vi "MIMIC_Test.vi"() -> ()   [LabVIEW 2014]
uses:
  Responses/MIMIC_ResponseCluster.ctl
panel:
  in  "Image":bool
  in  "Input_Data":string[](array[string])
  out "Generic_Mimic_Data":T1
  in  "Send":bool
  in  "Command":string
  in  "QUIT":bool
  in  "VISA_IN":refnum<visa-resource-name>="COM4"
  in  "Port Setting":T2={"baud rate"=9600, "data bits"=8, "parity (0:none)"=enum."None", "stop bits (10: 1 bit)"=10} {"stop bits (10: 1 bit)" items=["1.0"=10, "1.5"=15, "2.0"=20]; "data bits" min=5 max=8 step=1}
  out "Error_Out":errorcluster
  in  "Error_In":errorcluster
  # "LIST of Commands:\n1.- EnterFATMode\n2.- ExitFATMode\n3.- SendAck\n4.- StartSession\n5.- ImagerMode"
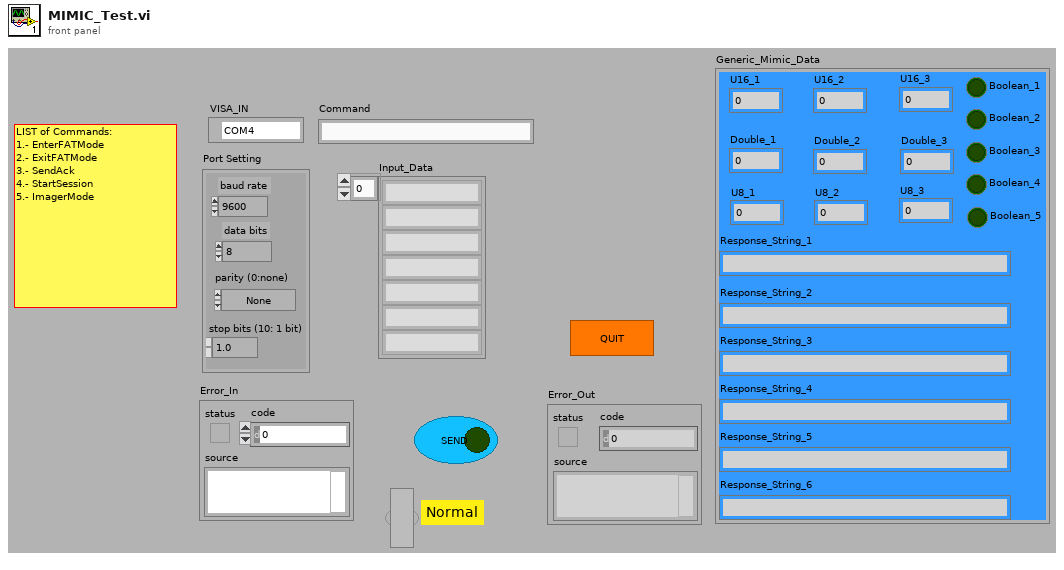
[diagram p1: front panel]
types:
  T1 = typedef "MIMIC_ResponseCluster.ctl" = cluster{"Response_String_1":string, "Response_String_2":string, "Response_String_3":string, "Response_String_4":string, "Response_String_5":string, "Response_String_6":string, "U16_1":u16, "Boolean_1":bool, "Boolean_2":bool, "Boolean_3":bool, "Boolean_4":bool, "Boolean_5":bool, "U16_2":u16, "U16_3":u16, "Double_1":dbl, "Double_2":dbl, "Double_3":dbl, "U8_1":dbl, "U8_2":dbl, "U8_3":dbl}
  T2 = cluster{"baud rate":u32, "data bits":u16, "parity (0:none)":enum16{"None", "Odd", "Even", "Mark", "Space"}, "stop bits (10: 1 bit)":u16}
  T3 = enum16{"OpenPort", "Initial Serial Port", "Write", "ByteRead", "Read", "ClearBuff", "Close"}
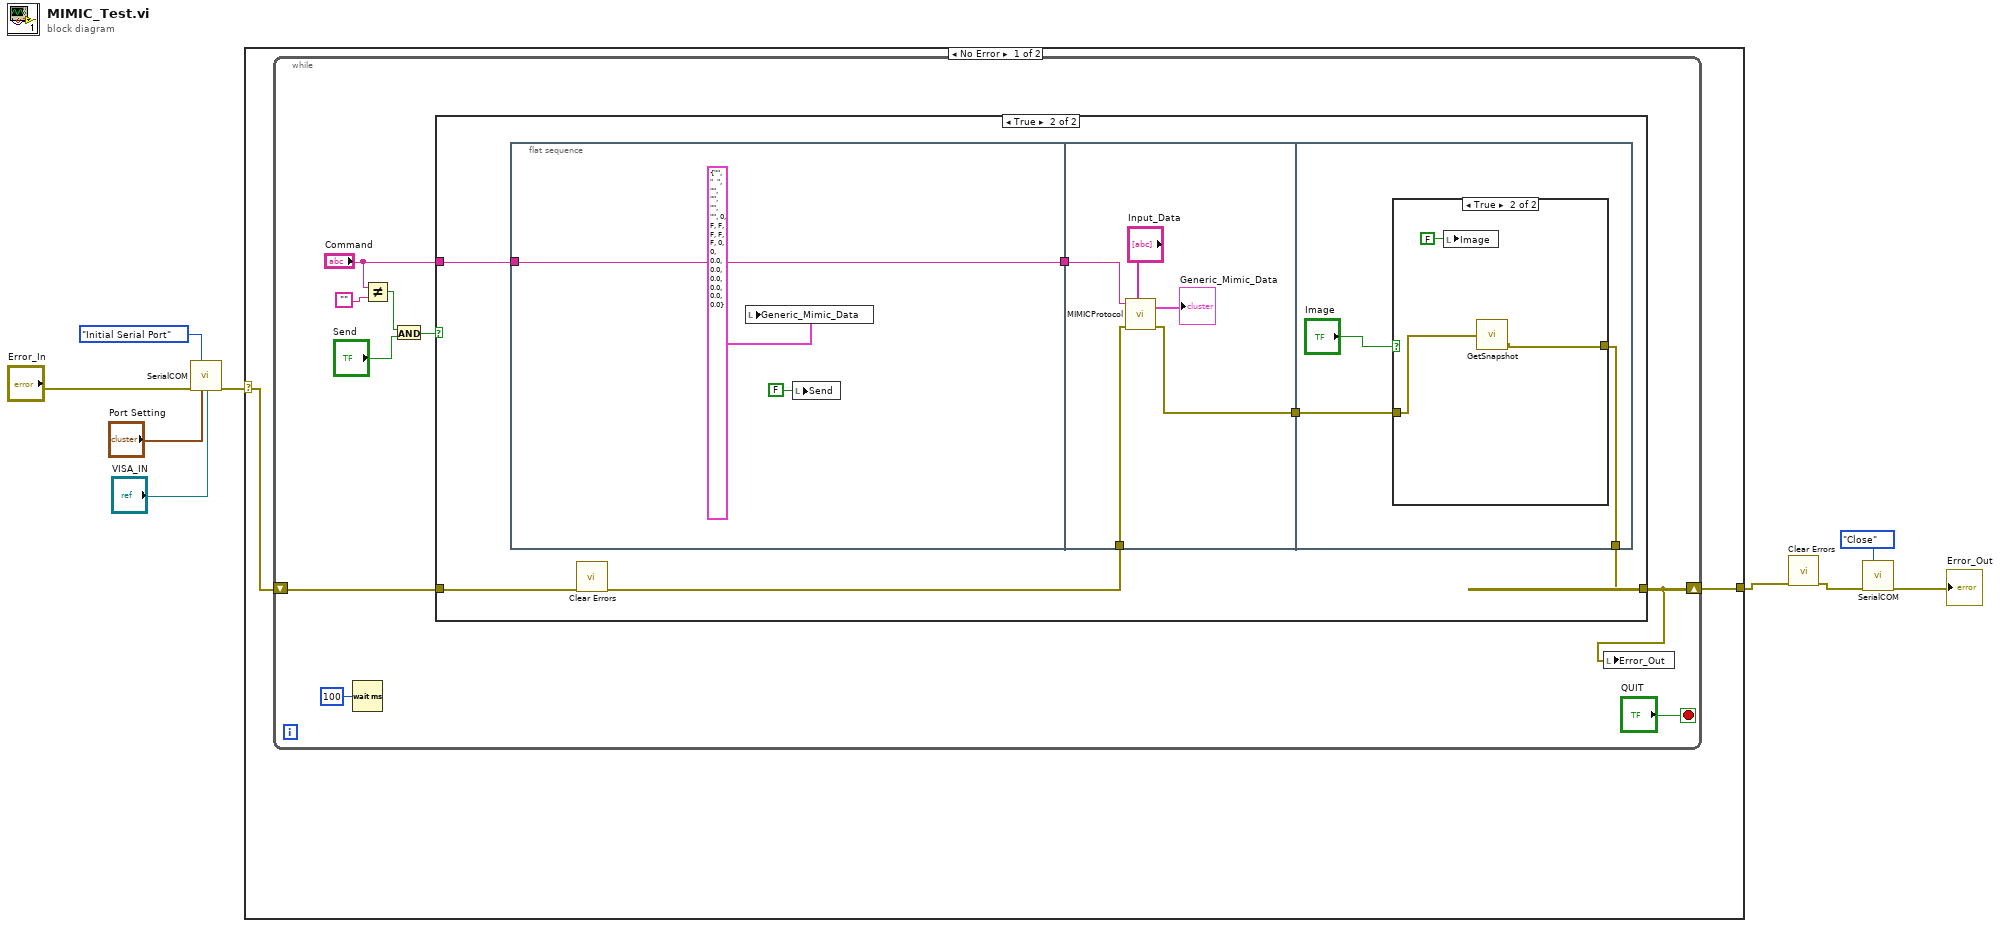
[diagram p0: block diagram]
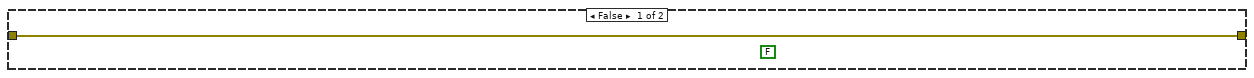
[diagram p2: hidden frame]
diagram:
  n1 = call "SerialCOM.vi"("Function"=T3."Initial Serial Port", "error in (no error)"="Error_In", "Port Setting"="Port Setting", "VISA_IN"="VISA_IN") -> ("error out"=w5:errorcluster)  [unwired: 6 in, 5 out]
  n2 = case shown="No Error" w5 {
    selector: w5 -> [w11 w43]
    tunnel: [w10 w43] -> w2
    frame No Error {
      n3 = while {
        shift-right: [w17] -> w10
        shift-left: w11 -> [w20]
        stop <- "QUIT" stop-if-true
        n4 = Wait (ms)(milliseconds to wait=u32 100) -> ()  [unwired: 1 out]
        n5 = Not Equal?(x="Command", y="") -> (x != y?=w14:bool)
        n6 = And(x=w14, y="Send") -> (x .and. y?=w12:bool)
        n7 = case shown="True" w12 {
          tunnel: w20 -> [w21 w25]
          tunnel: [w21 w22] -> w17
          tunnel: "Command" -> [_ w27]
          frame False {
            (unwired) FALSE
          }
          frame True {
            n8 = flat-sequence {
              tunnel: w27 -> [w30]
              tunnel: [w30] -> w26
              tunnel: w24 -> [w34]
              tunnel: w26 -> [w33]
              tunnel: [w31] -> w23
              tunnel: w23 -> [w37]
              tunnel: [w36] -> w22
              frame #0 {
                n9 = local write "Generic_Mimic_Data"(T1 {"Response_String_1"="", "Response_String_2"="  ", "Response_String_3"="", "Response_String_4"="", "Response_String_5"="", "Response_String_6"="", "U16_1"=0, "Boolean_1"=FALSE, "Boolean_2"=FALSE, "Boolean_3"=FALSE, "Boolean_4"=FALSE, "Boolean_5"=FALSE, "U16_2"=0, "U16_3"=0, "Double_1"=0.0, "Double_2"=0.0, "Double_3"=0.0, "U8_1"=0.0, "U8_2"=0.0, "U8_3"=0.0} ("Generic_Mimic_Data")) -> ()
                n10 = local write "Send"(FALSE ("Send")) -> ()
              }
              frame #1 {
                n11 = call "MIMICProtocol.vi"("Input_Data"="Input_Data", "Error In"=w34, "MIMIC_Command"=w33) -> ("Error Out"=w31:errorcluster, "Generic_Mimic_Data 2"=→"Generic_Mimic_Data":T1)  [unwired: 2 in, 2 out]
              }
              frame #2 {
                n12 = case shown="True" "Image" {
                  tunnel: w37 -> [w39 w41]
                  tunnel: [w39 w40] -> w36
                  frame False {
                  }
                  frame True {
                    n13 = local write "Image"(FALSE ("Image")) -> ()
                    n14 = call "GetSnapshot.vi"("error in"=w41) -> ("error out"=w40:errorcluster)  [unwired: 1 out]
                  }
                }
              }
            }
            n15 = call <vilib>:"Clear Errors.vi"("error in (no error)"=w25) -> ("error out"=w24:errorcluster)  [unwired: 5 in, 1 out]
          }
        }
        n16 = local write "Error_Out"(w17) -> ()
      }
    }
    frame Error {
    }
  }
  n17 = call <vilib>:"Clear Errors.vi"("error in (no error)"=w2) -> ("error out"=w1:errorcluster)  [unwired: 5 in, 1 out]
  n18 = call "SerialCOM.vi"("Function"=T3."Close", "error in (no error)"=w1) -> ("error out"=→"Error_Out":errorcluster)  [unwired: 8 in, 5 out]
